vi "GEvt-Set Source Filter Rules - v1.0.vi"(8 "Error in":errorcluster caption="Error in (no error)", 11 "Rules-v1":T1) -> (0 "Error out":errorcluster)   [LabVIEW 2020, in "Communicable State Machine.lvlib"]
uses:
  Communicable State Machine.lvlib
  _CSM_GlobalLog Filter Rules - v1.0.ctl
  _CSM_GlobalLog_MSG_TYPE.ctl
  _CSM_GlobalLog_STATE_TYPE.ctl
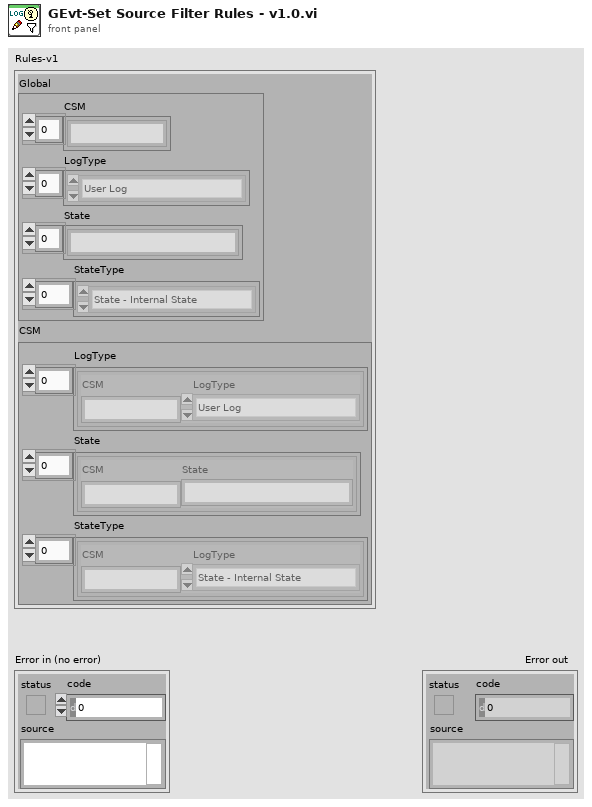
[diagram p1: front panel]
types:
  T1 = typedef "Communicable State Machine.lvlib/_CSM_GlobalLog Filter Rules - v1.0.ctl" = cluster{"Global":cluster{"CSM":string[], "LogType":T2[], "State":string[], "StateType":T3[]}, "CSM":cluster{"LogType":cluster{"CSM":string, "LogType":T2}[], "State":cluster{"CSM":string, "State":string}[], "StateType":cluster{"CSM":string, "LogType":T3}[]}}
  T2 = typedef "Communicable State Machine.lvlib/_CSM_GlobalLog_MSG_TYPE.ctl" = enum16{"User Log", "State Change", "Status", "Interrupt", "Register", "Unregister", "Error Log", "Module Created", "Module Destroyed"}
  T3 = typedef "Communicable State Machine.lvlib/_CSM_GlobalLog_STATE_TYPE.ctl" = enum16{"State - Internal State", "State - External Message", "State - Response", "State - Complete"}
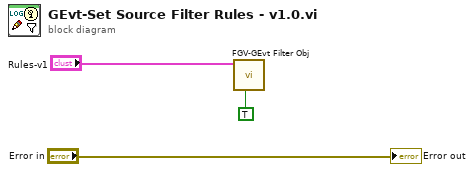
[diagram p0: block diagram]
diagram:
  n1 = call "FGV-GEvt Filter Obj.vi"("Set(T)/Get(F)"=TRUE, "Rules-v1"="Rules-v1") -> ()  [unwired: 8 in, 2 out]
  "Error out" <- "Error in"
